vi "Notify Observers (Event).vi"(8 "error in (no error)":errorcluster, 10 "Message":refnum<class "MSG.lvclass">, 11 "ObserverRegistry in":refnum<class "ObserverRegistry.lvclass">) -> (0 "error out":errorcluster, 3 "ObserverRegistry out":refnum<class "ObserverRegistry.lvclass">)   [LabVIEW 2011, in "Messenging.lvlib" / "ObserverRegistry.lvclass"]
uses:
  ObserverRegistry.lvclass
  Interprocess Messenger/TextVarientMessage/MSG.lvclass
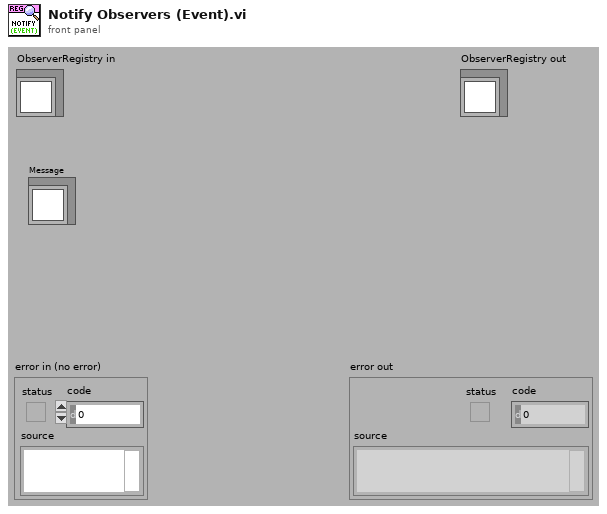
[diagram p1: front panel]
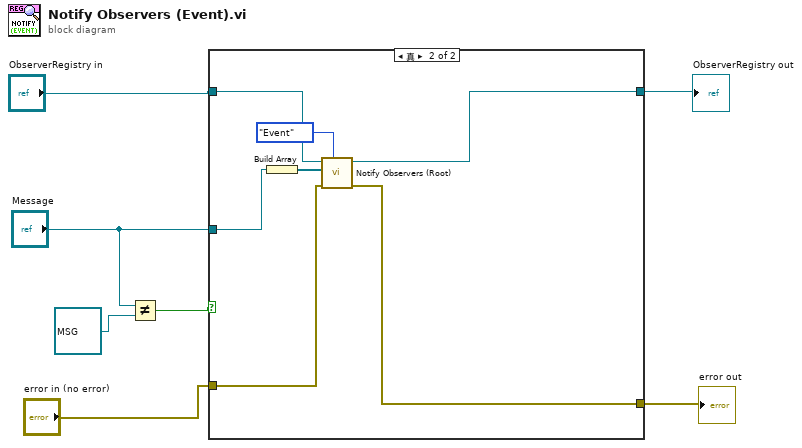
[diagram p0: block diagram]
diagram:
  n1 = Not Equal?(x="Message", y=refnum<class "MSG.lvclass"> refnum ("Message")) -> (x != y?=w4:bool)
  n2 = case shown="真" w4 {
    tunnel: "ObserverRegistry in" -> [w9 w16]
    tunnel: [w9 w13] -> w1
    tunnel: "error in (no error)" -> [w8 w12]
    tunnel: [w8 w11] -> w2
    tunnel: "Message" -> [_ w15]
    frame False {
      # "Null Message"
    }
    frame True {
      n3 = Build Array(w15) -> (w14:refnum<class "MSG.lvclass">[])
      n4 = call "Notify Observers (Root).vi"("Type"=enum16{"Event", "State"}."Event", "error in (no error)"=w12, "Array of State Messages"=w14, "ObserverRegistry in"=w16) -> ("error out"=w11:errorcluster, "ObserverRegistry out"=w13:refnum<class "ObserverRegistry.lvclass">)  [unwired: 6 out]
    }
  }
  "error out" <- w2
  "ObserverRegistry out" <- w1
